vi "PH_Powermeter_BaseClass.set wanted Setting to GUI.vi"(0 "VI in":refnum<vi>, 5 "error in (no error)":errorcluster) -> (14 "VI out":refnum<vi>, 19 "error out":errorcluster)   [LabVIEW 2014, in "PH_Powermeter_BaseClass.lvlib"]
uses:
  PH_Powermeter_BaseClass.lvlib
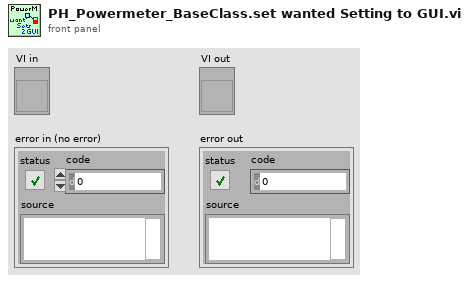
[diagram p1: front panel]
types:
  T1 = typedef "PH_Powermeter_BaseClass.lvlib/PH_Powermeter_BaseClass.i attribute.ctl" = cluster{"GUI References":T2, "Connection":T3, "Head Attributes":T5, "VISA resource":refnum<visa-resource-name>, "Energy":T6, "Service ID Energy":i32, "Wanted Settings":T7, "Current Settings":T7}
  T2 = typedef "PH_Powermeter_BaseClass.lvlib/PH_Powermeter_BaseClass.GUI Refs.ctl" = cluster{"Head Attributes":refnum<vi>, "Energy":refnum<vi>, "Connection":refnum<vi>, "VISA Resource":refnum<vi>, "Scaling Factor":refnum<vi>, "Range":refnum<vi>, "Wavelength":refnum<vi>, "Trigger Level":refnum<vi>, "Wanted Settings":refnum<vi>, "Current Settings":refnum<vi>}
  T3 = typedef "PH_Powermeter_BaseClass.lvlib/PH_Powermeter_BaseClass.Connection.ctl" = cluster{"failed checks":i8, "Timeout":bool, "Data read":string, "Failure":bool, "Error":bool, "State":T4}
  T4 = typedef "PH_Powermeter_BaseClass.lvlib/PH_Powermeter_BaseClass.State.ctl" = enum32{"off", "operating", "opened", "checked", "connected", "Sets to change", "running"}
  T5 = typedef "PH_Powermeter_BaseClass.lvlib/PH_Powermeter_BaseClass.Head Attributes.ctl" = cluster{"Instrument Type":string, "Head Version":string, "Head Name":string, "Serial Number":string, "Firmware":string, "Sensor Type":string, "MinimumRange":u32, "Maximum Range":u32, "Min Wavelength":i32, "Max Wavelength":i32}
  T6 = typedef "PH_Powermeter_BaseClass.lvlib/PH_Powermeter_BaseClass.Energy.ctl" = cluster{"current Value":dbl, "unscaled":dbl, "Scaling Factor":dbl}
  T7 = typedef "PH_Powermeter_BaseClass.lvlib/PH_gentec_BaseClass.Head Settings.ctl" = cluster{"Trigger Level":dbl, "Wavelength":u32, "Range":u32}
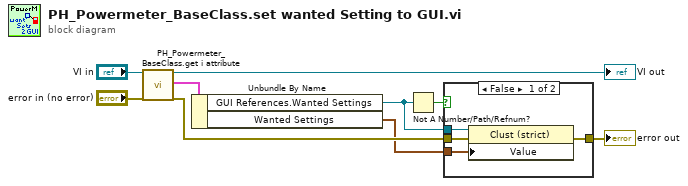
[diagram p0: block diagram]
diagram:
  n1 = call "PH_Powermeter_BaseClass.get i attribute.vi"("i ref in"="VI in", "error in (no error)"="error in (no error)") -> ("i ref out"=→"VI out":refnum<vi>, "i attribute"=w4:T1, "error out"=w9:errorcluster)  [unwired: 15 in]
  n2 = Unbundle By Name(w4) -> ("GUI References.Wanted Settings"=w1:refnum<vi>, "Wanted Settings"=w3:T7)
  n3 = Not A Number/Path/Refnum?(number/path/refnum=w1) -> (NaN/Path/Refnum?=w2:bool)
  n4 = case shown="False" w2 {
    tunnel: w9 -> [w13 w14]
    tunnel: [w12 w14] -> w5
    tunnel: w1 -> [w11 _]
    tunnel: w3 -> [w10 _]
    frame False {
      n5 = property class="Clust (strict)"(reference=w11, error in=w13, "Value"=w10) -> (error out=w12:errorcluster)  [unwired: 1 out]
    }
    frame True {
    }
  }
  "error out" <- w5
